vi "Get Next.vi"(0 "Loop in":refnum<class "Loop.lvclass">, 1 "Linked List Ref":refnum<data-value>, 5 "Active Unique ID":string, 9 "Active Element Index":i32, 11 "error in (no error)":errorcluster) -> (3 "Linked List Ref out":refnum<data-value>, 4 "Executioner out":refnum<class "Executioner.lvclass">, 6 "Active Unique ID out":string, 8 "Test Executive Ref out":refnum<data-value>, 10 "Active Element Index out":i32, 12 "Found":bool, 13 "Complete":bool, 14 "Stop":bool, 15 "error out":errorcluster)   [LabVIEW 2017, in "Custom Type Test Executive.lvlib" / "Loop.lvclass"]
uses:
  <vilib>/gpm_packages/@cs/test-executive/Source/Custom Type Test Executive/Loop/Loop.lvclass
  C:/Program Files/National Instruments/LabVIEW 2017/vi.lib/gpm_packages/@cs/test-executive/Source/Test Executive/Executioner/Executioner.lvclass
  <vilib>/gpm_packages/@cs/test-executive/Source/Test Executive/Executioner/Executioner.lvclass
  <vilib>/gpm_packages/@cs/linked-list/Source/Linked List/ILinkedList/ILinked List.lvclass
  <vilib>/gpm_packages/@cs/test-executive/Source/Test Executive/ITestExecutive/ITest Executive.lvclass
  <vilib>/gpm_packages/@cs/data-type-serializer/source/I32/I32.lvclass/I32.ctl
  <vilib>/gpm_packages/@cs/data-type-serializer/source/Boolean/Boolean.lvclass/Boolean.ctl
  a18d9f7e-17b5-481f-8f77-1e03f003462d.vi
  3009fa94-c7a9-4f4f-b9cc-2fa386d69e94.vi
  e0022fd2-631d-48e2-91bd-9c4263ef235c.vi
  11c1fdc4-8fc1-4fe4-90c3-e3ba1437ba00.vi
  a427ce06-9f36-467f-86ec-b3cc61723476.vi
  1adc3f9d-8519-4790-b64c-d8ab19fd0891.vi
  <vilib>/gpm_packages/@cs/data-type-serializer/source/I32/I32.lvclass
  C:/Program Files/National Instruments/LabVIEW 2017/vi.lib/gpm_packages/@cs/data-type-serializer/source/Data Type/Data Type.lvclass
  <vilib>/gpm_packages/@cs/data-type-serializer/source/Boolean/Boolean.lvclass
  <vilib>/gpm_packages/@cs/linked-list/Source/Linked List/Linked List Ref/Linked List Ref.lvclass
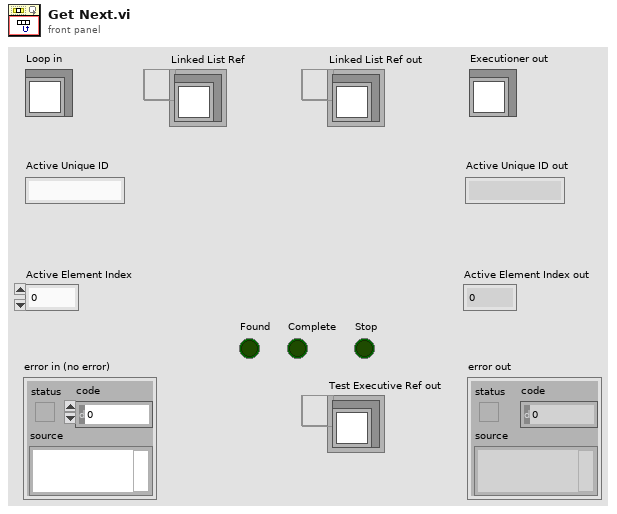
[diagram p1: front panel]
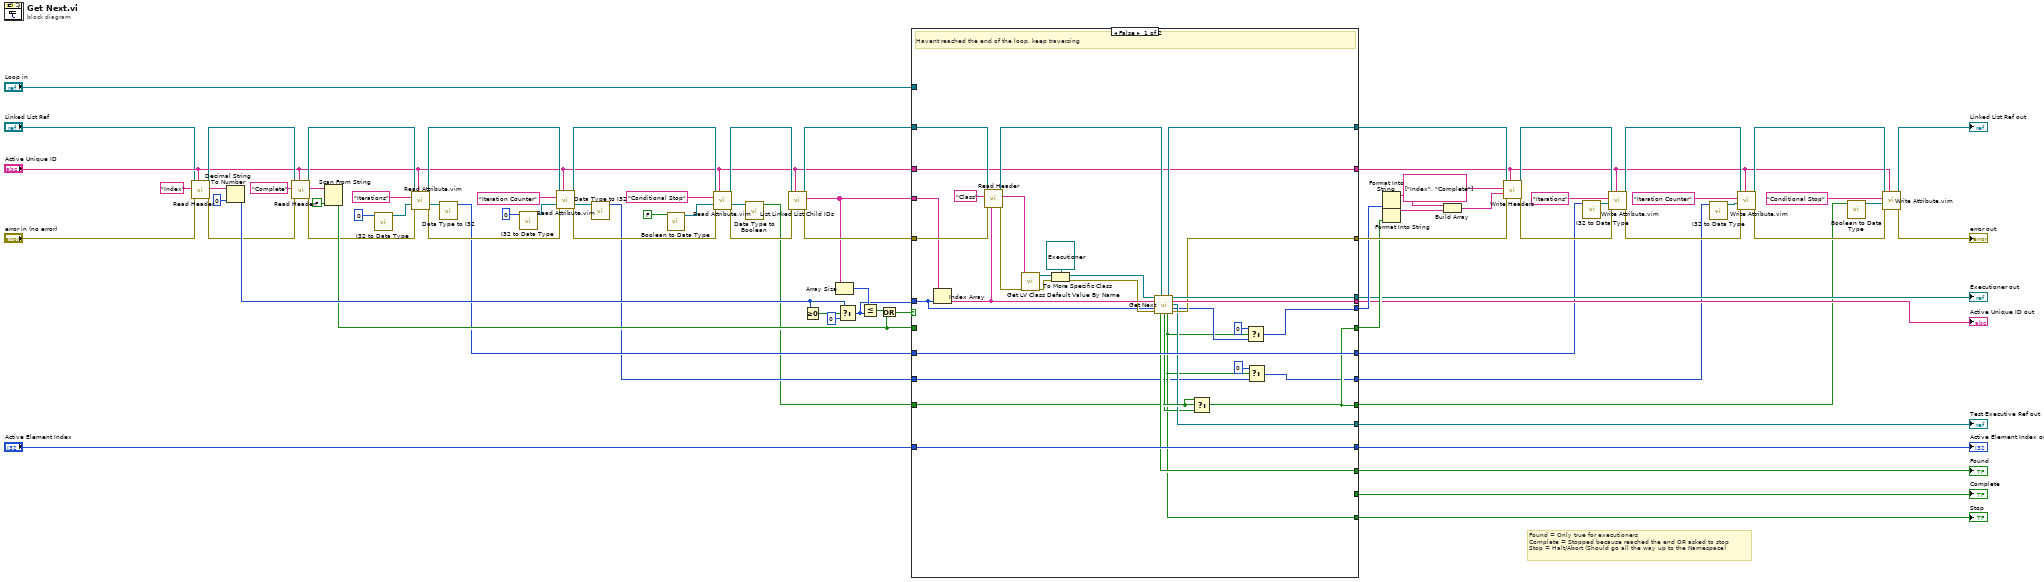
[diagram p0: block diagram]
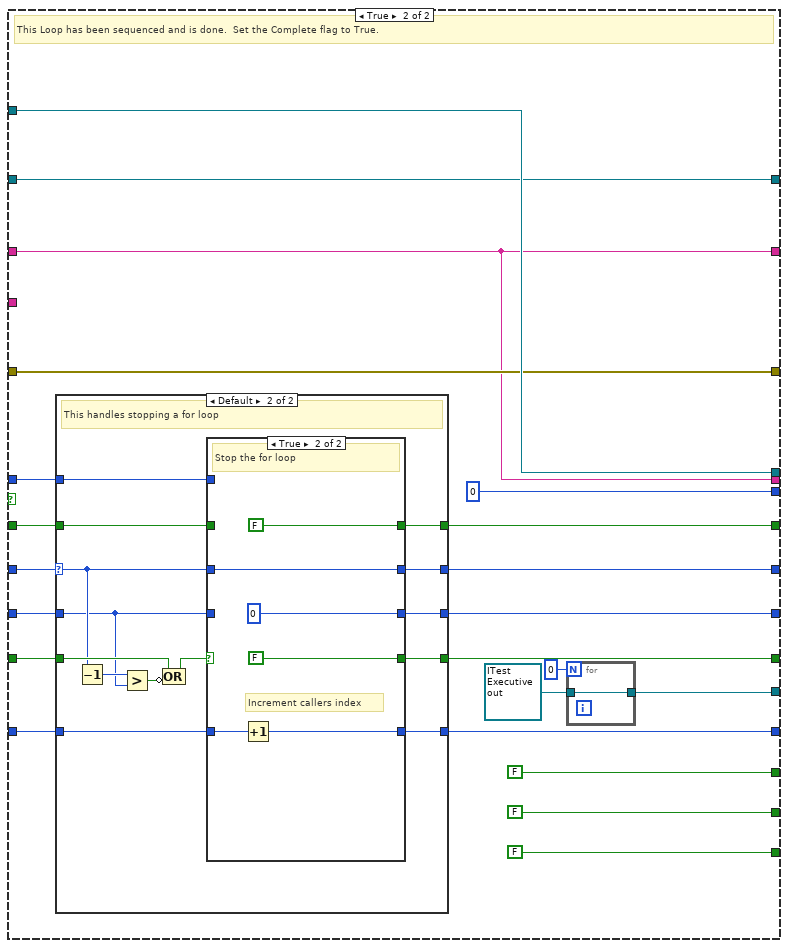
[diagram p2: hidden frame]
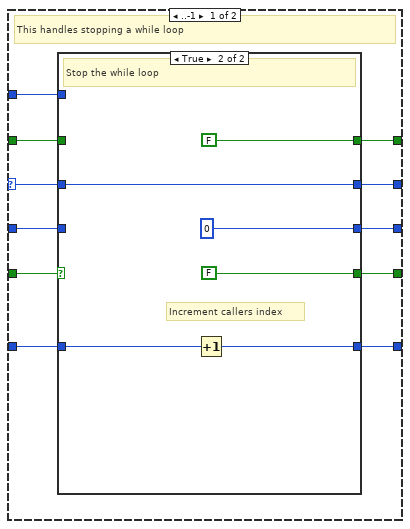
[diagram p3: hidden frame]
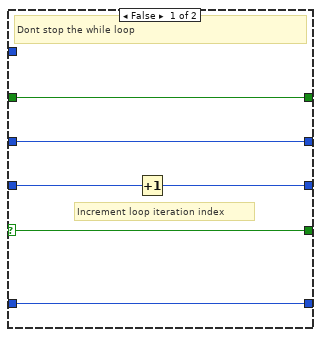
[diagram p4: hidden frame]
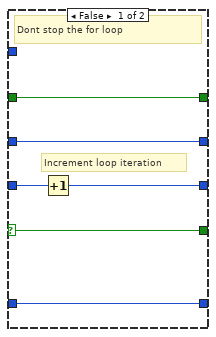
[diagram p5: hidden frame]
diagram:
  # "Found = Only true for executioners\nComplete = Stopped because reached the end OR asked to stop\nStop = Halt/Abort (Should go all the way up to the Namespace)"
  n1 = call <vilib>:"Read Header.vi"("Linked List ID"="Active Unique ID", "error in (no error)"="error in (no error)", "Header Name"="Index" ("Attribute Name"), "Linked List Ref"="Linked List Ref") -> ("error out"=w37:errorcluster, "Header Value"=w43:string, "Linked List Ref out"=w38:refnum<data-value>)  [unwired: 4 in, 1 out]
  n2 = Decimal String To Number(string=w43, default (0L)=0 ("Attribute")) -> (number=w72:i32)  [unwired: 1 in, 1 out]
  n3 = call <vilib>:"Read Header.vi"("Linked List ID"="Active Unique ID", "error in (no error)"=w37, "Header Name"="Complete" ("Attribute Name"), "Linked List Ref"=w38) -> ("error out"=w47:errorcluster, "Header Value"=w40:string, "Linked List Ref out"=w50:refnum<data-value>)  [unwired: 4 in, 1 out]
  n4 = Scan From String(input string=w40, default 1=FALSE) -> (output 1=w66:bool)  [unwired: 3 in, 3 out]
  n5 = call <vilib>:"I32 to Data Type.vi"("I32"=0) -> ("Boolean out"=w17:refnum<class "I32.lvclass">)  [unwired: 9 in, 1 out]
  n6 = call "Read Attribute.vim"("Linked List Ref"=w50, "Linked List ID"="Active Unique ID", "Attribute Name"="Iterations", "Type"=w17, "error in (no error)"=w47) -> ("Linked List Ref out"=w49:refnum<data-value>, "Attribute"=w16:refnum<class "I32.lvclass">, "error out"=w46:errorcluster)  [unwired: 5 in, 3 out]
  n7 = call <vilib>:"Data Type to I32.vi"("Data Type"=w16) -> ("I32 out"=w15:i32)  [unwired: 9 in, 1 out]
  n8 = call <vilib>:"I32 to Data Type.vi"("I32"=0) -> ("Boolean out"=w13:refnum<class "I32.lvclass">)  [unwired: 9 in, 1 out]
  n9 = call "Read Attribute.vim"("Linked List Ref"=w49, "Linked List ID"="Active Unique ID", "Attribute Name"="Iteration Counter", "Type"=w13, "error in (no error)"=w46) -> ("Linked List Ref out"=w58:refnum<data-value>, "Attribute"=w12:refnum<class "I32.lvclass">, "error out"=w57:errorcluster)  [unwired: 5 in, 3 out]
  n10 = call <vilib>:"Data Type to I32.vi"("Data Type"=w12) -> ("I32 out"=w11:i32)  [unwired: 9 in, 1 out]
  n11 = call <vilib>:"Boolean to Data Type.vi"("Boolean"=FALSE) -> ("Boolean out"=w10:refnum<class "Boolean.lvclass">)  [unwired: 9 in, 1 out]
  n12 = call "Read Attribute.vim"("Linked List Ref"=w58, "Linked List ID"="Active Unique ID", "Attribute Name"="Conditional Stop", "Type"=w10, "error in (no error)"=w57) -> ("Linked List Ref out"=w78:refnum<data-value>, "Attribute"=w8:refnum<class "Boolean.lvclass">, "error out"=w77:errorcluster)  [unwired: 5 in, 3 out]
  n13 = call <vilib>:"Data Type to Boolean.vi"("Data Type"=w8) -> ("Boolean out"=w7:bool)  [unwired: 9 in, 1 out]
  n14 = call <vilib>:"List Linked List Child IDs.vi"("Linked List ID"="Active Unique ID", "error in (no error)"=w77, "Linked List Ref"=w78) -> ("error out"=w70:errorcluster, "Child IDs"=w68:string[], "Linked List Ref out"=w71:refnum<data-value>)  [unwired: 6 in]
  n15 = Greater Or Equal To 0?(x=w72) -> (x >= 0?=w76:bool)
  n16 = Array Size(array=w68) -> (size(s)=w73:i32)
  n17 = Select(t=w72, s=w76, f=0) -> (s? t:f=w67:i32)
  n18 = Less Or Equal?(x=w73, y=w67) -> (x <= y?=w74:bool)
  n19 = Or(x=w74, y=w66) -> (x .or. y?=w69:bool)
  n20 = case shown="False" w69 {
    tunnel: w71 -> [w105 w133]
    tunnel: [w102 w133] -> w65
    tunnel: [w91 w134] -> w64
    tunnel: w70 -> [w104 w134]
    tunnel: w15 -> [w99 w129]
    tunnel: w11 -> [w82 w127]
    tunnel: w7 -> [w94 w128]
    tunnel: w68 -> [w101 _]
    tunnel: w67 -> [w100 w131]
    tunnel: [w99 w121] -> w5
    tunnel: [w81 w120] -> w3
    tunnel: [w85 0 ("Active Element Index out")] -> w63
    tunnel: [w98 w118] -> w21
    tunnel: [w97 w135] -> w20
    tunnel: "Loop in" -> [_ w135]
    tunnel: "Active Element Index" -> [w96 w126]
    tunnel: [w96 w123] -> w24
    tunnel: [_ FALSE] -> w26
    tunnel: [w83 FALSE] -> w27
    tunnel: "Active Unique ID" -> [w93 w118]
    tunnel: w66 -> [_ w130]
    tunnel: [w95 FALSE] -> w25
    tunnel: [w90 w122] -> w62
    tunnel: [w90 w119] -> w1
    tunnel: [w93 w118] -> w45
    tunnel: [w89 w115] -> w23
    frame False {
      # "Havent reached the end of the loop, keep traversing"
      n21 = Index Array(array=w101, index=w100) -> (element=w112:string)
      n22 = call <vilib>:"Read Header.vi"("Linked List ID"=w112, "error in (no error)"=w104, "Header Name"="Class", "Linked List Ref"=w105) -> ("error out"=w92:errorcluster, "Header Value"=w111:string, "Linked List Ref out"=w103:refnum<data-value>)  [unwired: 4 in, 1 out]
      n23 = call <vilib>:"Get LV Class Default Value By Name.vi"("error in (no error)"=w92, "class name"=w111) -> ("error out"=w107:errorcluster, "object"=w110:refnum<class>)  [unwired: 8 in]
      n24 = To More Specific Class(target class=refnum<class "Executioner.lvclass"> refnum ("Test Executive.lvlib:Executioner.lvclass"), reference=w110, error in=w107) -> (specific class reference=w106:refnum<class "Executioner.lvclass">, error out=w108:errorcluster)
      n25 = call-dynamic "Get Next.vi"("Executioner in"=w106, "Linked List Ref"=w103, "Active Unique ID"=w112, "Active Element Index"=w100, "error in (no error)"=w108) -> ("Linked List Ref out"=w102:refnum<data-value>, "Executioner out"=w97:refnum<class "Executioner.lvclass">, "Active Unique ID out"=w98:string, "Test Executive Ref out"=w89:refnum<data-value>, "Active Element Index out"=w86:i32, "Found"=w95:bool, "Complete"=w88:bool, "Stop"=w83:bool, "error out"=w91:errorcluster)  [unwired: 2 in]
      n26 = Select(t=w94, s=w94, f=w88) -> (s? t:f=w90:bool)
      n27 = Select(t=0, s=w83, f=w86) -> (s? t:f=w85:i32)
      n28 = Select(t=0, s=w83, f=w82) -> (s? t:f=w81:i32)
    }
    frame True {
      # "This Loop has been sequenced and is done.  Set the Complete flag to True."
      n29 = case shown="Default" w129 {
        selector: w129 -> [w143 w161]
        tunnel: w128 -> [w147 w163]
        tunnel: w127 -> [w142 w160]
        tunnel: [w146 w173] -> w123
        tunnel: w126 -> [w145 w172]
        tunnel: w131 -> [w139 w168]
        tunnel: [w144 w171] -> w121
        tunnel: [w141 w170] -> w119
        tunnel: [w140 w169] -> w120
        tunnel: [w138 w167] -> w122
        tunnel: w130 -> [w137 w166]
        frame ..-1 {
          # "This handles stopping a while loop"
          n30 = case shown="True" w147 {
            selector: w147 -> [w149 _]
            tunnel: [w153 w158] -> w146
            tunnel: w145 -> [w153 w159]
            tunnel: [w150 w157] -> w144
            tunnel: w143 -> [w150 w157]
            tunnel: w142 -> [w152 _]
            tunnel: [w149 FALSE] -> w141
            tunnel: [w151 0 ("Numeric")] -> w140
            tunnel: w139 -> [_ _]
            tunnel: [w148 FALSE] -> w138
            tunnel: w137 -> [w148 _]
            frame False {
              # "Increment loop iteration index"
              # "Dont stop the while loop"
              n31 = Increment(x=w152) -> (x+1=w151:i32)
            }
            frame True {
              # "Increment callers index"
              # "Stop the while loop"
              n32 = Increment(x=w159) -> (x+1=w158:i32)
            }
          }
        }
        frame Default {
          # "This handles stopping a for loop"
          n33 = Decrement(x=w161) -> (x-1=w165:i32)
          n34 = Greater?(x=w165, y=w160) -> (0:w164:bool)
          n35 = Compound Arithmetic op=OR(w163, invert w164) -> (w162:bool)
          n36 = case shown="True" w162 {
            selector: w162 -> [w175 _]
            tunnel: [w179 w184] -> w173
            tunnel: w172 -> [w179 w185]
            tunnel: [w176 w183] -> w171
            tunnel: w161 -> [w176 w183]
            tunnel: w160 -> [w178 _]
            tunnel: [w175 FALSE] -> w170
            tunnel: [w177 0 ("Numeric")] -> w169
            tunnel: w168 -> [_ _]
            tunnel: [w174 FALSE] -> w167
            tunnel: w166 -> [w174 _]
            frame False {
              # "Increment loop iteration"
              # "Dont stop the for loop"
              n37 = Increment(x=w178) -> (x+1=w177:i32)
            }
            frame True {
              # "Increment callers index"
              # "Stop the for loop"
              n38 = Increment(x=w185) -> (x+1=w184:i32)
            }
          }
        }
      }
      n39 = for {
        N: 0 -> [_]
        tunnel: refnum<data-value> refnum ("Test Executive Ref out") -> [w136]
        tunnel: [w136] -> w115
      }
    }
  }
  "Executioner out" <- w20
  "Active Unique ID out" <- w21
  "Active Element Index out" <- w24
  "Found" <- w25
  "Complete" <- w26
  "Stop" <- w27
  "Test Executive Ref out" <- w23
  n40 = Format Into String(w63) -> (resulting string=w35:string)  [unwired: 3 in, 1 out]
  n41 = Format Into String(w62) -> (resulting string=w34:string)  [unwired: 3 in, 1 out]
  n42 = Build Array(w35, w34) -> (w33:string[])
  n43 = call <vilib>:"Write Headers.vi"("Linked List ID"=w45, "error in (no error)"=w64, "Header Values"=w33, "Header Names"=string[] ["Index", "Complete"], "Linked List Ref"=w65) -> ("error out"=w60:errorcluster, "Linked List Ref out"=w59:refnum<data-value>)  [unwired: 5 in]
  n44 = call <vilib>:"I32 to Data Type.vi"("I32"=w5) -> ("Boolean out"=w6:refnum<class "I32.lvclass">)  [unwired: 9 in, 1 out]
  n45 = call "Write Attribute.vim"("Linked List ID"=w45, "error in (no error)"=w60, "Attribute"=w6, "Attribute Name"="Iterations", "Linked List Ref"=w59) -> ("error out"=w55:errorcluster, "Linked List Ref out"=w56:refnum<data-value>)  [unwired: 3 in, 2 out]
  n46 = call <vilib>:"I32 to Data Type.vi"("I32"=w3) -> ("Boolean out"=w4:refnum<class "I32.lvclass">)  [unwired: 9 in, 1 out]
  n47 = call "Write Attribute.vim"("Linked List ID"=w45, "error in (no error)"=w55, "Attribute"=w4, "Attribute Name"="Iteration Counter", "Linked List Ref"=w56) -> ("error out"=w52:errorcluster, "Linked List Ref out"=w53:refnum<data-value>)  [unwired: 3 in, 2 out]
  n48 = call <vilib>:"Boolean to Data Type.vi"("Boolean"=w1) -> ("Boolean out"=w2:refnum<class "Boolean.lvclass">)  [unwired: 9 in, 1 out]
  n49 = call "Write Attribute.vim"("Linked List ID"=w45, "error in (no error)"=w52, "Attribute"=w2, "Attribute Name"="Conditional Stop", "Linked List Ref"=w53) -> ("error out"=→"error out":errorcluster, "Linked List Ref out"=→"Linked List Ref out":refnum<data-value>)  [unwired: 3 in, 2 out]
